vi "GetWaveform.vi"(0 "Acq ID Out":u32, 1 "Read Mode":enum32{"ADC", "Volts"}(ring), 5 "Num Samps":i32=1000, 9 "Num Segs":i32, 11 "error in":errorcluster, 12 "Channel":i32=1) -> (3 "Dig Word Size":u16, 4 "Acq ID Out":u32, 6 "Acquired Waveform SGL":dbl[][](array[numeric]), 8 "Acquired Waveform16 bit":i16[][](array[numeric]), 10 "first row":dbl[](array[numeric]) format="%.2f", 13 "segDescArray out":T2(array[cluster]) {"horPos" format="%.3e"}, 14 "dataDesc":T1 {"reserved3" format="%.3e"; "vOffset" format="%.2f"; "vGain" format="%.2e"; "sampTime" format="%.3e"}, 15 "error out":errorcluster)   [LabVIEW 2022 SP3]
uses:
  <instrlib>/Acqiris Dx/Public/Data/Read Multi-Segments I8.vi
  <instrlib>/Acqiris Dx/Public/Data/Read Multi-Segments I16.vi
  <instrlib>/Acqiris Dx/Public/Data/Read Multi-Segments DBL.vi
  <instrlib>/Acqiris Bx/Acqiris Bx.lvlib
  <instrlib>/Acqiris Dx/Acqiris Dx.lvlib
panel:
  # "Mujst convert data at output for Integers"
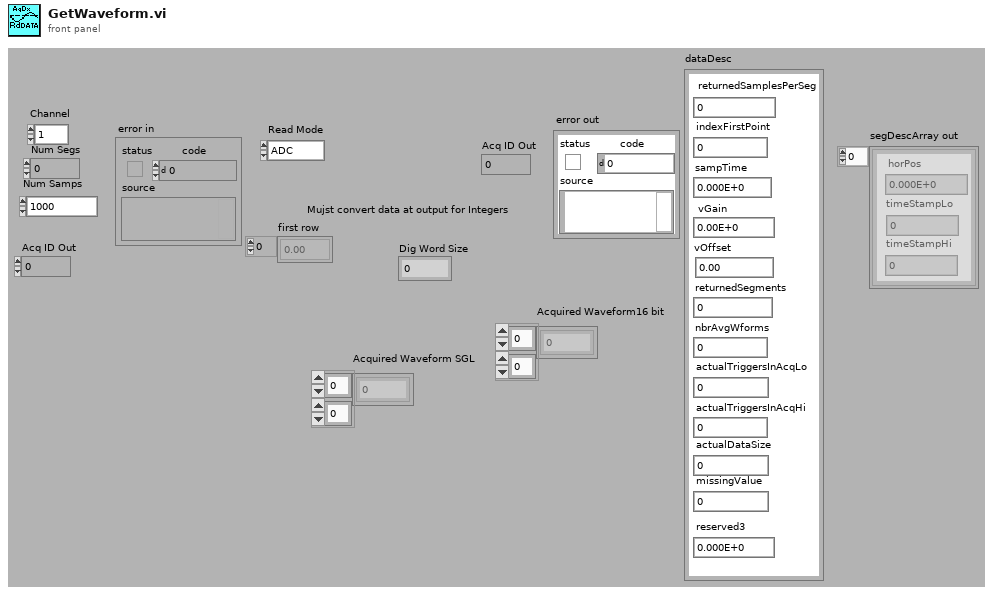
[diagram p1: front panel]
types:
  T1 = cluster{"returnedSamplesPerSeg":i32, "indexFirstPoint":i32, "sampTime":dbl, "vGain":dbl, "vOffset":dbl, "returnedSegments":i32, "nbrAvgWforms":i32, "actualTriggersInAcqLo":u32, "actualTriggersInAcqHi":u32, "reserved3":dbl, "actualDataSize":u32, "missingValue":dbl}
  T2 = cluster{"horPos":dbl, "timeStampLo":u32, "timeStampHi":u32}[]
  T3 = cluster{"dataType":i32, "readMode":i32, "firstSegment":i32, "nbrSegments":i32, "firstSampleInSeg":i32, "nbrSamplesInSeg":i32, "segmentOffset":i32, "dataArraySize":i32, "segDescArraySize":i32, "flags":i32, "reserved2":dbl, "reserved3":dbl, "reserved":i32}
  T4 = cluster{"horPos":dbl, "timeStampLo":u32, "timeStampHi":u32}
  T5 = cluster{"returnedSamplesPerSeg":i32, "indexFirstPoint":i32, "sampTime":dbl, "vGain":dbl, "vOffset":dbl, "returnedSegments":i32, "nbrAvgWforms":i32, "actualTriggersInAcqLo":u32, "actualTriggersInAcqHi":u32, "actualDataSize":u32, "missingValue":i32, "reserved3":dbl}
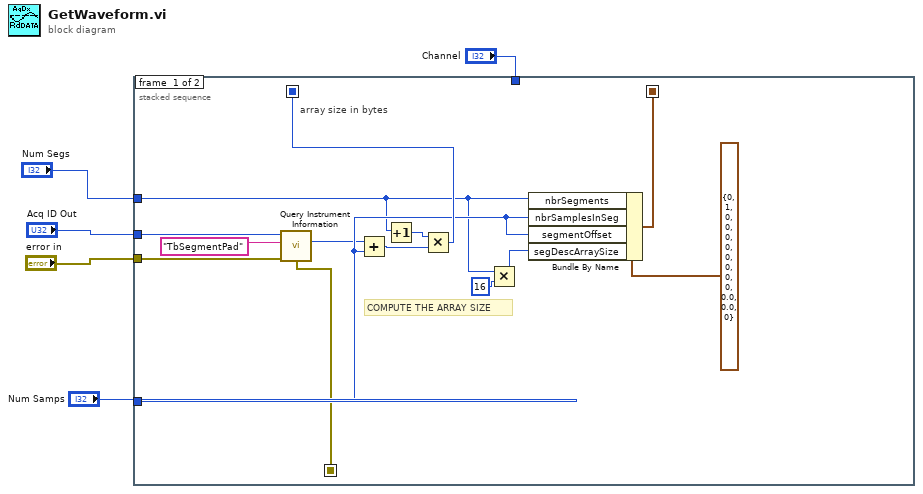
[diagram p0: block diagram]
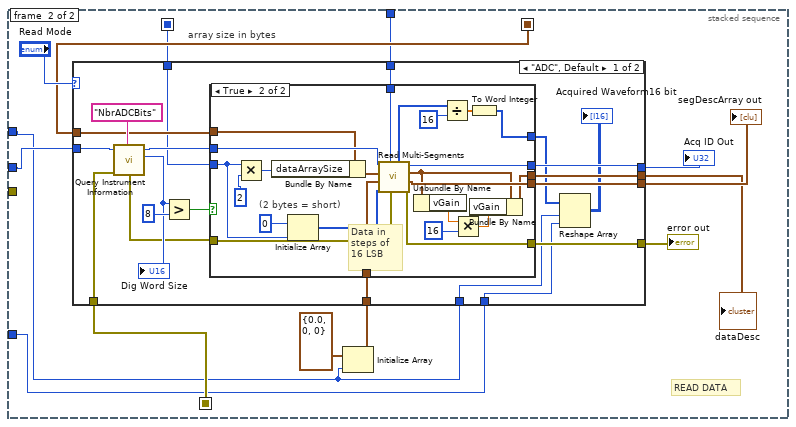
[diagram p2: hidden frame]
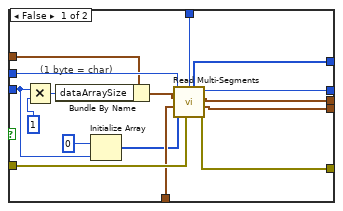
[diagram p3: hidden frame]
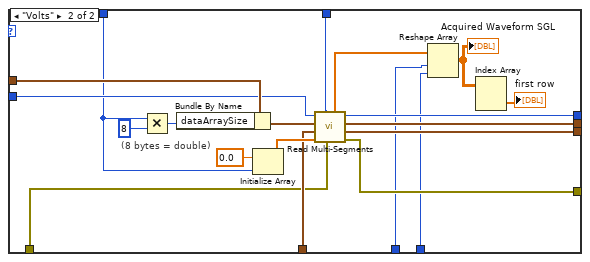
[diagram p4: hidden frame]
diagram:
  n1 = stacked-sequence {
    seq-local: [w7 _] -> [_ w28]
    seq-local: [w12 _] -> [_ w26]
    seq-local: [w11 _] -> [_ w25]
    tunnel: "error in" -> [w14 _]
    tunnel: "Acq ID Out" -> [w13 w27]
    tunnel: "Num Samps" -> [w10 w21]
    tunnel: "Num Segs" -> [w9 w20]
    tunnel: "Channel" -> [_ w23]
    frame #0 {
      # "COMPUTE THE ARRAY SIZE"
      # "array size in bytes"
      n2 = call <instrlib>:"Query Instrument Information.vi"("Instrument ID"=w13, "Parameter String"="TbSegmentPad", "error in (no error)"=w14) -> ("Info Value (I32)"=w8:i32, "error out"=w7:errorcluster)  [unwired: 1 in, 4 out]
      n3 = Add(x=w8, y=w10) -> (x+y=w16:i32)
      n4 = Increment(x=w9) -> (x+1=w17:i32)
      n5 = Multiply(x=w17, y=w16) -> (x*y=w11:i32)
      n6 = Multiply(x=w9, y=16) -> (x*y=w19:i32)
      n7 = Bundle By Name(cluster=T3 {"dataType"=0, "readMode"=1, "firstSegment"=0, "nbrSegments"=0, "firstSampleInSeg"=0, "nbrSamplesInSeg"=0, "segmentOffset"=0, "dataArraySize"=0, "segDescArraySize"=0, "flags"=0, "reserved2"=0.0, "reserved3"=0.0, "reserved"=0} ("readPar"), "nbrSegments"=w9, "nbrSamplesInSeg"=w10, "segmentOffset"=w10, "segDescArraySize"=w19) -> (w12:T3)
    }
    frame #1 {
      # "READ DATA"
      # "array size in bytes"
      n8 = Initialize Array(T4 {"horPos"=0.0, "timeStampLo"=0, "timeStampHi"=0} ("cluster"), w20) -> (w31:T2)
      n9 = case shown="\"ADC\", Default" "Read Mode" {
        tunnel: w26 -> [w44 w108]
        tunnel: w31 -> [w48 w110]
        tunnel: w25 -> [w42 w99]
        tunnel: w27 -> [w47 w107]
        tunnel: [w50 w106] -> w32
        tunnel: [w51 w105] -> w22
        tunnel: [w52 w104] -> w33
        tunnel: [w49 w103] -> w24
        tunnel: w23 -> [w43 w102]
        tunnel: w28 -> [w45 w101]
        tunnel: w21 -> [w37 w96]
        tunnel: w20 -> [w36 w95]
        frame "ADC", Default {
          n10 = call <instrlib>:"Query Instrument Information.vi"("Instrument ID"=w47, "Parameter String"="NbrADCBits", "error in (no error)"=w45) -> ("dup Instrument ID"=w46:u32, "Info Value (I32)"=w39:i32, "error out"=w38:errorcluster)  [unwired: 1 in, 3 out]
          "Dig Word Size" <- w39
          n11 = Greater?(x=w39, y=8) -> (0:w41:bool)
          n12 = case shown="True" w41 {
            tunnel: [w54 w91] -> w52
            tunnel: [w68 w74] -> w51
            tunnel: [w67 w90] -> w50
            tunnel: [w55 w89] -> w49
            tunnel: w38 -> [w66 w88]
            tunnel: [w65 w71] -> w35
            tunnel: w43 -> [w64 w87]
            tunnel: w46 -> [w63 w86]
            tunnel: w48 -> [w62 w85]
            tunnel: w44 -> [w59 w82]
            tunnel: w42 -> [w57 w80]
            frame False {
              # "(1 byte = char)"
              n13 = Multiply(x=w57, y=1) -> (x*y=w60:i32)
              n14 = Bundle By Name(cluster=w59, "dataArraySize"=w60) -> (w58:T3)
              n15 = Initialize Array(i8 0 ("element"), w57) -> (w61:i8[])
              n16 = call-poly <instrlib>:"Read Multi-Segments.vi"("error in (no error)"=w66, "channel"=w64, "dataArray in"=w61, "segDescArray in"=w62, "readPar"=w58, "Instrument ID"=w63) -> ("error out"=w55:errorcluster, "segDescArray out"=w67:T2, "dataDesc"=w68:T5, "dup Instrument ID"=w54:u32, "dataArray out"=w65:i8[])
            }
            frame True {
              # "Data in steps of 16 LSB"
              # "(2 bytes = short)"
              n17 = Multiply(x=w80, y=2) -> (x*y=w83:i32)
              n18 = Bundle By Name(cluster=w82, "dataArraySize"=w83) -> (w81:T3)
              n19 = Initialize Array(i16 0 ("element"), w80) -> (w84:i16[])
              n20 = call-poly <instrlib>:"Read Multi-Segments.vi"("error in (no error)"=w88, "channel"=w87, "dataArray in"=w84, "segDescArray in"=w85, "readPar"=w81, "Instrument ID"=w86) -> ("error out"=w89:errorcluster, "segDescArray out"=w90:T2, "dataDesc"=w78:T5, "dup Instrument ID"=w91:u32, "dataArray out"=w72:i16[])
              n21 = Unbundle By Name(w78) -> ("vGain"=w76:dbl)
              n22 = Divide(x=w72, y=16) -> (x/y=w70:dbl[])
              n23 = Multiply(x=w76, y=16) -> (x*y=w75:dbl)
              n24 = To Word Integer(number=w70) -> (16bit integer=w71:i16[])
              n25 = Bundle By Name(cluster=w78, "vGain"=w75) -> (w74:T5)
            }
          }
          n26 = Reshape Array(w35, w36, w37) -> (→"Acquired Waveform16 bit":i16[][])
        }
        frame "Volts" {
          # "(8 bytes = double)"
          n27 = Multiply(x=w99, y=8) -> (x*y=w100:i32)
          n28 = Bundle By Name(cluster=w108, "dataArraySize"=w100) -> (w109:T3)
          n29 = Initialize Array(0.0 ("element"), w99) -> (w111:dbl[])
          n30 = call-poly <instrlib>:"Read Multi-Segments.vi"("error in (no error)"=w101, "channel"=w102, "dataArray in"=w111, "segDescArray in"=w110, "readPar"=w109, "Instrument ID"=w107) -> ("error out"=w103:errorcluster, "segDescArray out"=w106:T2, "dataDesc"=w105:T5, "dup Instrument ID"=w104:u32, "dataArray out"=w97:dbl[])
          n31 = Reshape Array(w97, w95, w96) -> (w94:dbl[][])
          "Acquired Waveform SGL" <- w94
          n32 = Index Array(array=w94) -> (element=→"first row":dbl[])  [unwired: 2 in]
        }
      }
      "segDescArray out" <- w32
      "error out" <- w24
      "Acq ID Out" <- w33
      "dataDesc" <- w22
    }
  }
